vi "Write to File.vi"(8 "error in (no error)":errorcluster, 10 "INI Ref":T1, 11 "Mouse Action in":refnum<class "Mouse Action.lvclass">) -> (0 "error out":errorcluster, 2 "INI Ref out":T1, 3 "Mouse Action out":refnum<class "Mouse Action.lvclass">)   [LabVIEW 2020, in "MacroAssert.lvlib" / "Mouse Action.lvclass"]
uses:
  Mouse Action.lvclass
  Mouse Action.lvclass/Mouse Action.ctl
  Action Step/Action Step.lvclass
  MacroAssert.lvlib
  <vilib>/Utility/config.llb/NI_LVConfig.lvlib
  <vilib>/Utility/config.llb/Write Key (I32).vi
  <vilib>/Utility/config.llb/Write Key (String).vi
  <vilib>/Utility/config.llb/Write Key (Boolean).vi
  <vilib>/Utility/config.llb/Config Data RefNum.ctl
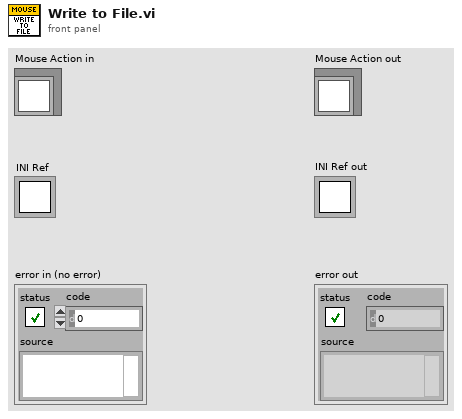
[diagram p1: front panel]
types:
  T1 = typedef "NI_LVConfig.lvlib/Config Data RefNum.ctl" = refnum<k1>
  T2 = typedef "MacroAssert.lvlib/Mouse Action.lvclass/Relative Movement Type.ctl" = enum16{"Pixels from Current Position", "Pixels from Top-Left of Control", "Pixels from Top-Left of Window", "Percentage from Top-Left of Control", "Percentage from Top-Left of Window", "Percentage from Top-Left of Screen"}
  T3 = typedef "MacroAssert.lvlib/Mouse Action.lvclass/Click Type.ctl" = enum16{"Normal", "Hold", "Release"}
  T4 = typedef "MacroAssert.lvlib/Mouse Action.lvclass/Mouse Action Type.ctl" = enum16{"Click", "Absolute Move", "Absolute Move and Click", "Relative Move", "Relative Move and Click", "Wheel Up", "Wheel Down"}
  T5 = typedef "MacroAssert.lvlib/Mouse Action.lvclass/Button.ctl" = enum16{"Left", "Right", "Middle"}
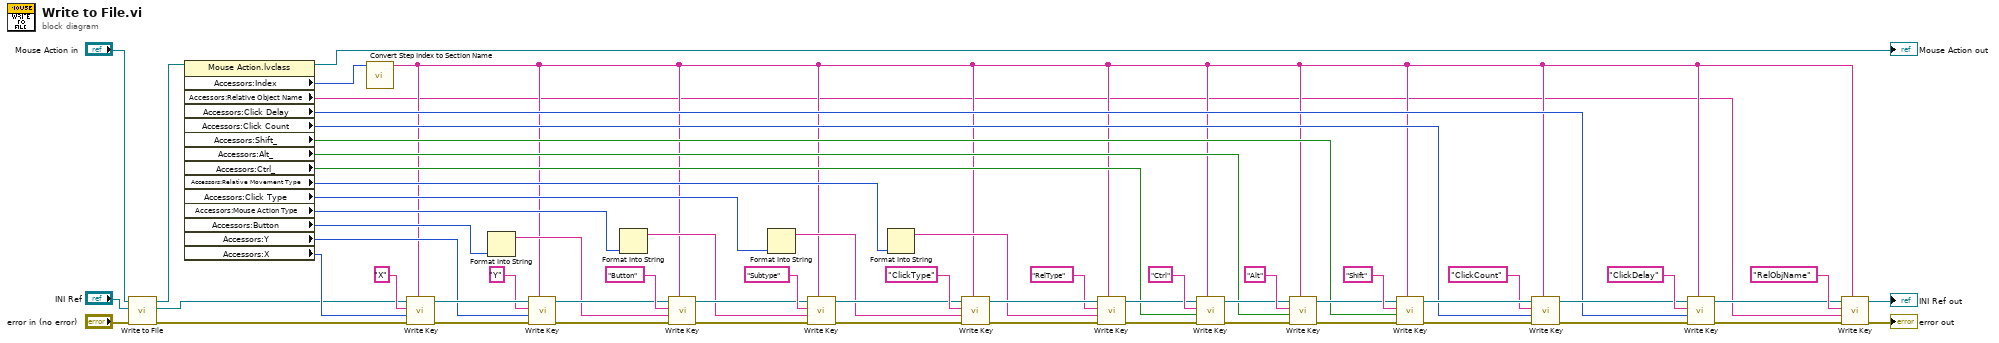
[diagram p0: block diagram]
diagram:
  n1 = call-parent "Write to File.vi"("error in (no error)"="error in (no error)", "INI Ref"="INI Ref", "Action Step in"="Mouse Action in") -> ("error out"=w52:errorcluster, "INI Ref out"=w49:T1, "Action Step out"=w51:refnum<class "Mouse Action.lvclass">)  [unwired: 6 in]
  n2 = property class="Mouse Action.lvclass"(reference=w51) -> (reference out=→"Mouse Action out":refnum<class "Mouse Action.lvclass">, "Accessors:Index"=w8:i32, "Accessors:Relative Object Name"=w1:string, "Accessors:Click Delay"=w9:i32, "Accessors:Click Count"=w10:i32, "Accessors:Shift_"=w11:bool, "Accessors:Alt_"=w12:bool, "Accessors:Ctrl_"=w13:bool, "Accessors:Relative Movement Type"=w30:T2, "Accessors:Click Type"=w32:T3, "Accessors:Mouse Action Type"=w36:T4, "Accessors:Button"=w34:T5, "Accessors:Y"=w53:i32, "Accessors:X"=w54:i32)  [unwired: 1 in, 1 out]
  n3 = call "Convert Step Index to Section Name.vi"("Step Index"=w8) -> ("Section Name"=w2:string)  [unwired: 10 in]
  n4 = call-poly <vilib>:"Write Key.vi"("section"=w2, "error in (no error)"=w52, "value"=w54, "key"="X", "refnum"=w49) -> ("error out"=w56:errorcluster, "refnum out"=w58:T1)  [unwired: 4 in, 1 out]
  n5 = Format Into String(w34) -> (resulting string=w33:string)  [unwired: 3 in, 1 out]
  n6 = call-poly <vilib>:"Write Key.vi"("section"=w2, "error in (no error)"=w56, "value"=w53, "key"="Y", "refnum"=w58) -> ("error out"=w47:errorcluster, "refnum out"=w46:T1)  [unwired: 4 in, 1 out]
  n7 = Format Into String(w36) -> (resulting string=w35:string)  [unwired: 3 in, 1 out]
  n8 = call-poly <vilib>:"Write Key.vi"("section"=w2, "error in (no error)"=w47, "value"=w33, "key"="Button", "refnum"=w46) -> ("error out"=w38:errorcluster, "refnum out"=w37:T1)  [unwired: 4 in, 1 out]
  n9 = Format Into String(w32) -> (resulting string=w31:string)  [unwired: 3 in, 1 out]
  n10 = call-poly <vilib>:"Write Key.vi"("section"=w2, "error in (no error)"=w38, "value"=w35, "key"="Subtype", "refnum"=w37) -> ("error out"=w41:errorcluster, "refnum out"=w39:T1)  [unwired: 4 in, 1 out]
  n11 = Format Into String(w30) -> (resulting string=w29:string)  [unwired: 3 in, 1 out]
  n12 = call-poly <vilib>:"Write Key.vi"("section"=w2, "error in (no error)"=w41, "value"=w31, "key"="ClickType", "refnum"=w39) -> ("error out"=w44:errorcluster, "refnum out"=w45:T1)  [unwired: 4 in, 1 out]
  n13 = call-poly <vilib>:"Write Key.vi"("section"=w2, "error in (no error)"=w44, "value"=w29, "key"="RelType", "refnum"=w45) -> ("error out"=w19:errorcluster, "refnum out"=w18:T1)  [unwired: 4 in, 1 out]
  n14 = call-poly <vilib>:"Write Key.vi"("section"=w2, "error in (no error)"=w19, "value"=w13, "key"="Ctrl", "refnum"=w18) -> ("error out"=w26:errorcluster, "refnum out"=w25:T1)  [unwired: 4 in, 1 out]
  n15 = call-poly <vilib>:"Write Key.vi"("section"=w2, "error in (no error)"=w26, "value"=w12, "key"="Alt", "refnum"=w25) -> ("error out"=w16:errorcluster, "refnum out"=w17:T1)  [unwired: 4 in, 1 out]
  n16 = call-poly <vilib>:"Write Key.vi"("section"=w2, "error in (no error)"=w16, "value"=w11, "key"="Shift", "refnum"=w17) -> ("error out"=w23:errorcluster, "refnum out"=w24:T1)  [unwired: 4 in, 1 out]
  n17 = call-poly <vilib>:"Write Key.vi"("section"=w2, "error in (no error)"=w23, "value"=w10, "key"="ClickCount", "refnum"=w24) -> ("error out"=w14:errorcluster, "refnum out"=w15:T1)  [unwired: 4 in, 1 out]
  n18 = call-poly <vilib>:"Write Key.vi"("section"=w2, "error in (no error)"=w14, "value"=w9, "key"="ClickDelay", "refnum"=w15) -> ("error out"=w6:errorcluster, "refnum out"=w5:T1)  [unwired: 4 in, 1 out]
  n19 = call-poly <vilib>:"Write Key.vi"("section"=w2, "error in (no error)"=w6, "value"=w1, "key"="RelObjName", "refnum"=w5) -> ("error out"=→"error out":errorcluster, "refnum out"=→"INI Ref out":T1)  [unwired: 4 in, 1 out]
